vi "Player Info.vi"(11 "DaveT in":refnum<class "DaveT.lvclass">) -> (0 "Defeat Speech":string, 1 "Victory Speech":string, 2 "Name":string, 3 "DaveT out":refnum<class "DaveT.lvclass">)   [LabVIEW 2017, in "DaveT.lvclass"]
uses:
  DaveT.lvclass
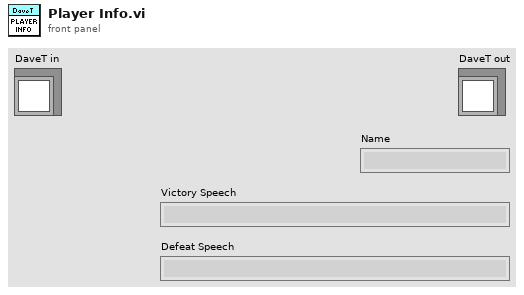
[diagram p1: front panel]
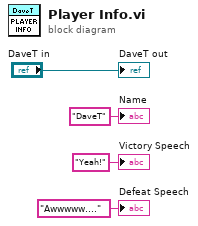
[diagram p0: block diagram]
diagram:
  "DaveT out" <- "DaveT in"
  "Name" <- "DaveT" ("Name")
  "Victory Speech" <- "Yeah!" ("Victory Speech")
  "Defeat Speech" <- "Awwwww...." ("Defeat Speech")
